vi "EncoderPositionControl.vi"() -> ()   [LabVIEW 2010]
uses:
  <vilib>/NXT/Subs/LVHSConnector.ctl
  <vilib>/NXT/NXTIO Xnodes/AddressXNode/NXTIOAddress.xnode
  <vilib>/NXT/Subs/MotorXNode.DC Motor Type.ctl
  <vilib>/NXT/Subs/MotorXNode.1DCMotor.ctl
  <vilib>/NXT/Subs/MotorXNode.2DCMotor.ctl
  <vilib>/NXT/NXTIO Xnodes/NXTIOXNode/NXTIO.xnode
  <vilib>/NXT/Dual Mode Library/Display/drawNumber.vi
  <vilib>/NXT/Dual Mode Library/Waits/Wait_Num(msec).vi
  <vilib>/NXT/NXTIO Xnodes/NXTIONodeSubVIs/TETRIX IO Reset Encoders.vi
  <vilib>/NXT/NXTIO Xnodes/NXTIONodeSubVIs/TETRIX IO Motor Status.vi
  <vilib>/NXT/NXTIO Xnodes/NXTIONodeSubVIs/TETRIX IO Move DC Motors.vi
  <vilib>/NXT/NXTIO Xnodes/NXTIONodeSubVIs/TETRIX IO Stop DC Motors.vi
panel:
  out "Enabled":bool
  out "iter":i32
  out "NXT":T1={"Hardware"="NXT", "Flattened String"=""}
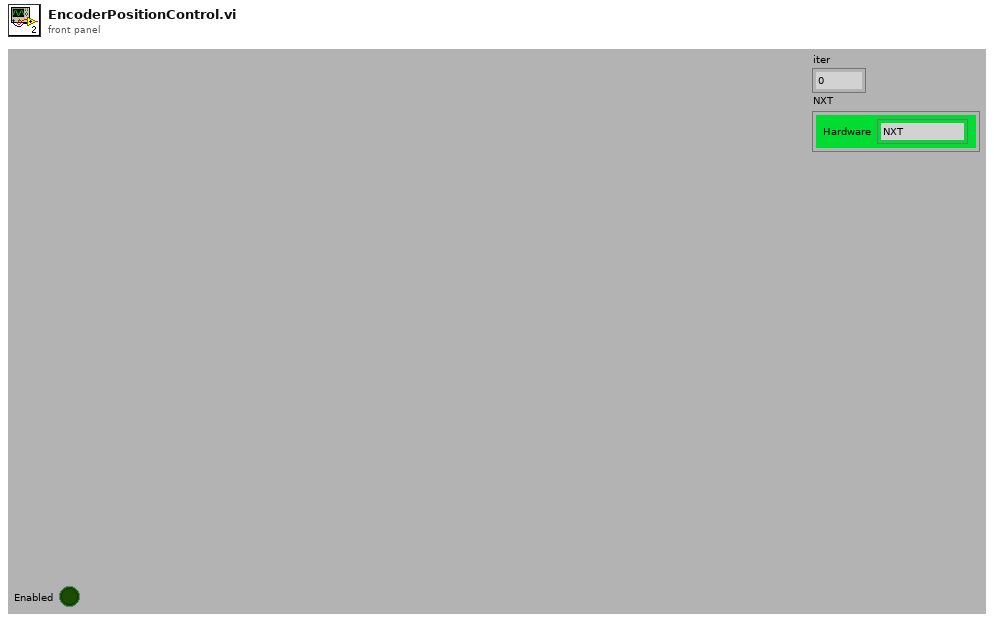
[diagram p1: front panel]
types:
  T1 = typedef "LVHSConnector.ctl" = cluster{"Hardware":string, "Flattened String":string}
  T2 = typedef "MotorXNode.DC Motor Type.ctl" = enum16{"DC Motor"}
  T3 = cluster{"DC Motor":T2, "Address":i16, "Address":i16}
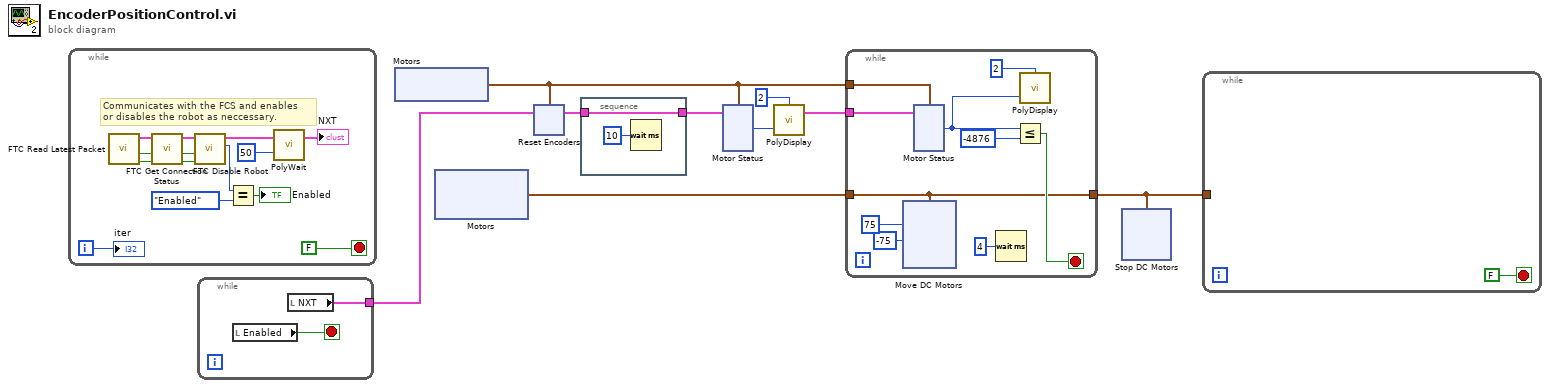
[diagram p0: block diagram]
diagram:
  n1 = while {
    i -> [w10]
    stop <- FALSE stop-if-true
    # "Communicates with the FCS and enables \nor disables the robot as neccessary."
    n2 = call <vilib>:"FTC Read Latest Packet.vi"() -> ("Packet Received?"=w21:bool, "Stopped?"=w20:bool, "NXT"=w23:T1)  [unwired: 6 in, 3 out]
    n3 = call <vilib>:"FTC Get Connection Status.vi"("Packet Received?"=w21, "Stopped?"=w20, "NXT"=w23) -> ("Online?"=w13:bool, "Stopped?"=w14:bool, "NXT"=w22:T1)  [unwired: 5 in]
    n4 = call <vilib>:"FTC Disable Robot.vi"("Online?"=w13, "Stopped?"=w14, "NXT"=w22) -> ("Enabled?"=w17:enum16{"Disabled", "Enabled"}, "NXT"=w19:T1)  [unwired: 3 in]
    n5 = Equal?(x=w17, y=enum16{"Disabled", "Enabled"}."Enabled") -> (x = y?=→"Enabled":bool)
    n6 = call-poly <vilib>:"PolyWait.vi"("Time (100 msec)"=u32 50 ("Time (msec)"), "NXT"=w19) -> ("NXT"=→"NXT":T1)  [unwired: 2 in]
    "iter" <- w10
  }
  n7 = while {
    tunnel: [w24] -> w8
    stop <- w25 stop-if-true
    n8 = local read "Enabled"() -> (w25:bool)
    n9 = local read "NXT"() -> (w24:T1)
  }
  n10 = xnode "Motors"() -> ("DC Motor"=w1:cluster{"DC Motor":T2, "Address":i16})
  n11 = xnode "Motors"() -> ("DC Motor"=w9:T3)
  n12 = xnode "Reset Encoders"("Motors"=w1, "NXT"=w8) -> ("NXT"=w6:T1)
  n13 = stacked-sequence {
    tunnel: w6 -> [w27]
    tunnel: [w27] -> w3
    frame #0 {
      n14 = Wait (ms)(milliseconds to wait=u32 10) -> ()  [unwired: 1 out]
    }
  }
  n15 = xnode "Motor Status"("Motors"=w1, "NXT"=w3) -> ("Position 1"=w4:i32)  [unwired: 2 out]
  n16 = call-poly <vilib>:"PolyDisplay.vi"("number"=w4, "Line"=2) -> ("NXT"=w2:T1)  [unwired: 2 in]
  n17 = while {
    tunnel: w2 -> [w36]
    tunnel: w9 -> [w33]
    tunnel: [w33] -> w7
    tunnel: w1 -> [w32]
    stop <- w35 stop-if-true
    n18 = xnode "Move DC Motors"("Power/Speed 2"=i8 -75, "Power/Speed 1"=i8 75 ("Power"), "Motors"=w33) -> ()  [unwired: 1 in, 1 out]
    n19 = xnode "Motor Status"("Motors"=w32, "NXT"=w36) -> ("Position 1"=w30:i32)  [unwired: 2 out]
    n20 = Wait (ms)(milliseconds to wait=u32 4) -> ()  [unwired: 1 out]
    n21 = Less Or Equal?(x=w30, y=-4876 ("Position")) -> (x <= y?=w35:bool)
    n22 = call-poly <vilib>:"PolyDisplay.vi"("number"=w30, "Line"=2) -> ()  [unwired: 2 in, 1 out]
  }
  n23 = xnode "Stop DC Motors"("Motors"=w7) -> ()  [unwired: 1 in, 1 out]
  n24 = while {
    tunnel: w7 -> [_]
    stop <- FALSE stop-if-true
  }
